vi "화12조 Data3.vi"(8 "error in":errorcluster caption="에러 입력") -> (0 "error out":errorcluster caption="에러 출력", 3 "task out":refnum<k21> caption="태스크 출력")   [LabVIEW 2020]
uses:
  <vilib>/DAQmx/create/channels.llb/DAQmx Create Channel (DI-Digital Input).vi
  <resource>/objmgr/daqmx.rc
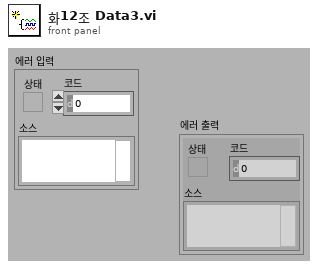
[diagram p1: front panel]
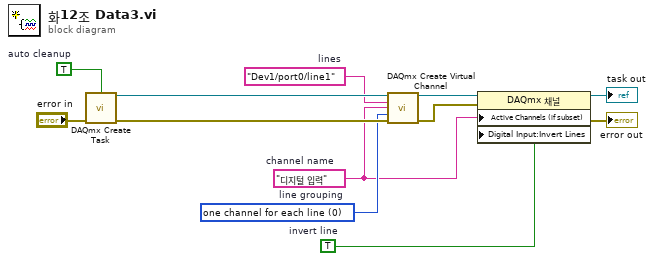
[diagram p0: block diagram]
diagram:
  w2 = TRUE  # invert line
  w7 = 0 items=["one channel for each line", "one channel for all lines"]  # line grouping
  w1 = "디지털 입력"  # channel name
  w8 = "Dev1/port0/line1"  # lines
  w10 = TRUE  # auto cleanup
  n1 = call <vilib>:"DAQmx Create Task.vi"("auto cleanup"=w10, "error in"="error in") -> ("task out"=w9:refnum<k21>, "error out"=w11:errorcluster)  [unwired: 12 in]
  n2 = call-poly <vilib>:"DAQmx Create Virtual Channel.vi"("task in"=w9, "lines"=w8, "name to assign"=w1, "line grouping"=w7, "error in"=w11) -> ("task out"=w6:refnum<k21>, "error out"=w5:errorcluster)  [unwired: 9 in]
  n3 = property class="DAQmx 채널"(reference=w6, error in=w5, "Active Channels (if subset)"=w1, "Digital Input:Invert Lines"=w2) -> (reference out=→"task out":refnum<k21>, error out=→"error out":errorcluster)
